vi "uw2u.vi"(2 "error in (no error)":errorcluster, 3 "uw":dbl) -> (0 "error out":errorcluster, 1 "u":dbl)   [LabVIEW 2021]
panel:
  out "J":dbl
  out "b":dbl
  out "CD":dbl
  out "Vin":dbl=15.54
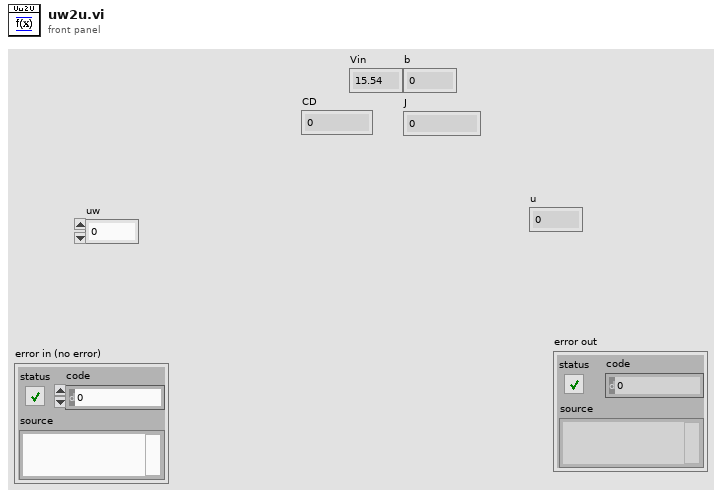
[diagram p1: front panel]
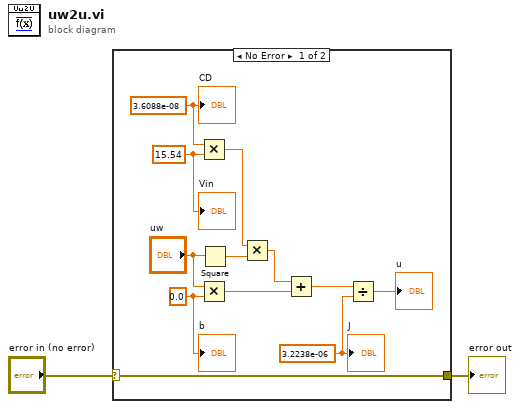
[diagram p0: block diagram]
diagram:
  n1 = case shown="No Error" "error in (no error)" {
    selector: "error in (no error)" -> [w14 w15]
    tunnel: [w14 w15] -> w1
    frame No Error {
      w4 = 3.2238e-06 ("y")
      w8 = 0.0 ("y")
      w10 = 15.54 ("y")
      w11 = 3.6088e-08 ("x")
      n2 = Multiply(x=w11, y=w10) -> (x*y=w12:dbl)
      n3 = Multiply(x="uw", y=w8) -> (x*y=w6:dbl)
      n4 = Square(x="uw") -> (x^2=w13:dbl)
      n5 = Multiply(x=w12, y=w13) -> (x*y=w7:dbl)
      n6 = Add(x=w7, y=w6) -> (x+y=w5:dbl)
      n7 = Divide(x=w5, y=w4) -> (x/y=→"u":dbl)
      "Vin" <- w10
      "CD" <- w11
      "b" <- w8
      "J" <- w4
    }
    frame Error {
    }
  }
  "error out" <- w1
